vi "CondBinner.vi"(0 "input":dbl) -> (1 "FrequencyIndex":i32, 2 "test13_version":string="C")   [LabVIEW 2019]
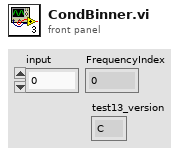
[diagram p1: front panel]
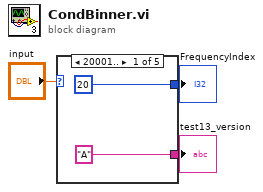
[diagram p0: block diagram]
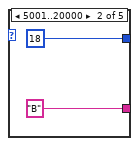
[diagram p2: hidden frame]
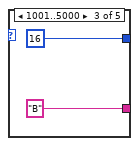
[diagram p3: hidden frame]
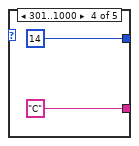
[diagram p4: hidden frame]
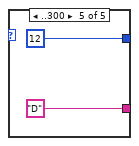
[diagram p5: hidden frame]
diagram:
  n1 = case shown="20001.." "input" {
    tunnel: [20 18 16 14 12] -> w2
    tunnel: ["A" "B" "B" "C" "D"] -> w1
    frame 20001.. {
    }
    frame 5001..20000 {
    }
    frame 1001..5000 {
    }
    frame 301..1000 {
    }
    frame ..300 {
    }
  }
  "FrequencyIndex" <- w2
  "test13_version" <- w1
